vi "createEngine.vi"(8 "error in (no error)":errorcluster, 9 "uiControlsMgr.lvclass":refnum<class "uiControlsMgr.lvclass">, 11 "Simon_Engine in":refnum<class "Simon_Engine.lvclass">) -> (0 "error out":errorcluster, 3 "Simon_Engine out":refnum<class "Simon_Engine.lvclass">)   [LabVIEW 2019, in "Simon_Engine.lvclass"]
doc: "Builds a new Simon Engine."
uses:
  Simon_Engine.lvclass
  uiControlsMgr/uiControlsMgr.lvclass
  Simon_Engine.lvclass/Simon_Engine.ctl
  LED/LED Class/LED.lvclass
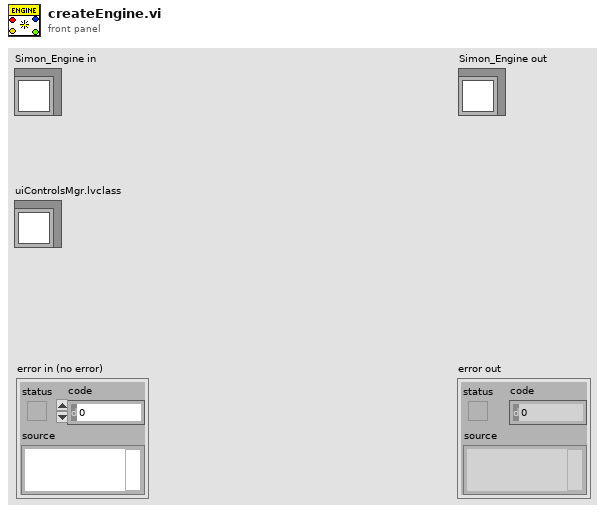
[diagram p1: front panel]
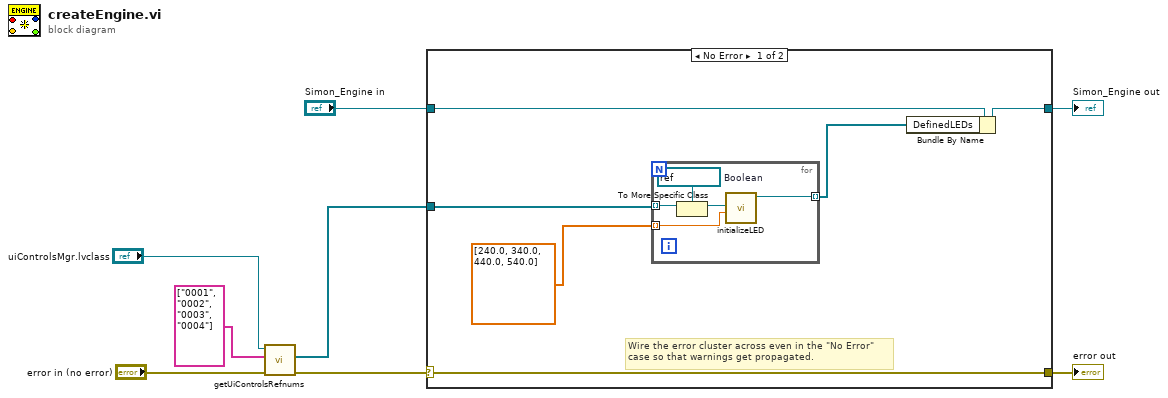
[diagram p0: block diagram]
diagram:
  n1 = call "getUiControlsRefnums.vi"("error in (no error)"="error in (no error)", "Control Indexes"=string[] ["0001", "0002", "0003", "0004"], "uiControlsMgr in"="uiControlsMgr.lvclass") -> ("error out"=w4:errorcluster, "Control Refnums"=w2:refnum<vi>[])  [unwired: 6 in, 1 out]
  n2 = case shown="No Error" w4 {
    selector: w4 -> [w13 w21]
    tunnel: [w13 w21] -> w7
    tunnel: [w12 w20] -> w5
    tunnel: "Simon_Engine in" -> [w14 w20]
    tunnel: w2 -> [w10 _]
    frame No Error {
      # "Wire the error cluster across even in the \"No Error\"\ncase so that warnings get propagated."
      n3 = for {
        tunnel: [w19] -> w11 mode=indexing
        tunnel: w10 -> [w18] mode=indexing
        tunnel: dbl[] [240.0, 340.0, 440.0, 540.0] -> [w17] mode=indexing
        w15 = refnum<vi> refnum  # Boolean
        n4 = To More Specific Class(target class=w15, reference=w18) -> (specific class reference=w16:refnum<vi>)  [unwired: 1 in, 1 out]
        n5 = call "initializeLED.vi"("frequency"=w17, "LED Refnum"=w16) -> ("LED out"=w19:refnum<class "LED.lvclass">)  [unwired: 8 in, 1 out]
      }
      n6 = Bundle By Name(cluster=w14, "DefinedLEDs"=w11) -> (w12:refnum<class "Simon_Engine.lvclass">)
    }
    frame Error {
    }
  }
  "error out" <- w7
  "Simon_Engine out" <- w5
